vi "Configure Front Panel View.vi"(8 "error in":errorcluster, 10 "Show All":bool, 11 "Heat Flow Test Stand in":refnum<class "Heat Flow Test Stand.lvclass">) -> (0 "error out":errorcluster, 3 "Heat Flow Test Stand out":refnum<class "Heat Flow Test Stand.lvclass">)   [LabVIEW 2019, in "Test Stands.lvlib" / "Heat Flow Test Stand.lvclass"]
uses:
  Heat Flow Test Stand.lvclass
  Generic Test Stand/TS Panel Method.ctl
  Generic Test Stand/Generic Test Stand.lvclass
  Results/Results Method.ctl
  Results/Results.lvlib
  Results/DeepU Results/DeepU Results.lvclass
  DAC/DAC.lvclass
  Results/Heat Flow Results/Heat Flow Results.lvclass
  C:/Users/krio/Documents/LV_Projects/test-stand/App/Generic Test Stand/Generic Test Stand.lvclass
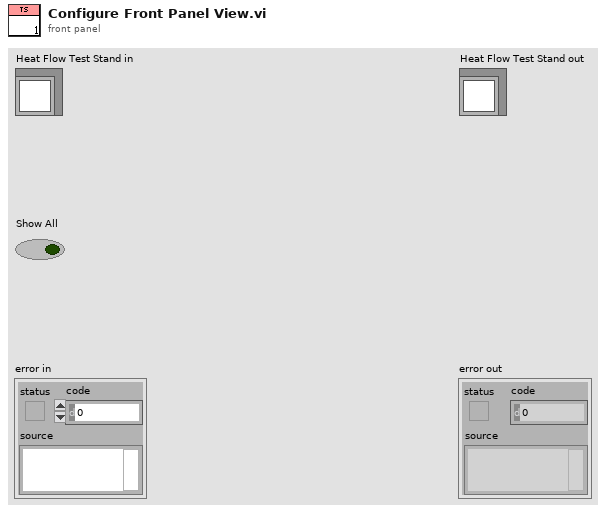
[diagram p1: front panel]
types:
  T1 = typedef "Generic Test Stand.lvclass/TS Panel Method.ctl" = enum16{"Send to Panel", "Receive from Panel", "Update Panel View"}
  T2 = typedef "Results.lvlib/Results Method.ctl" = enum16{"Get", "Set"}
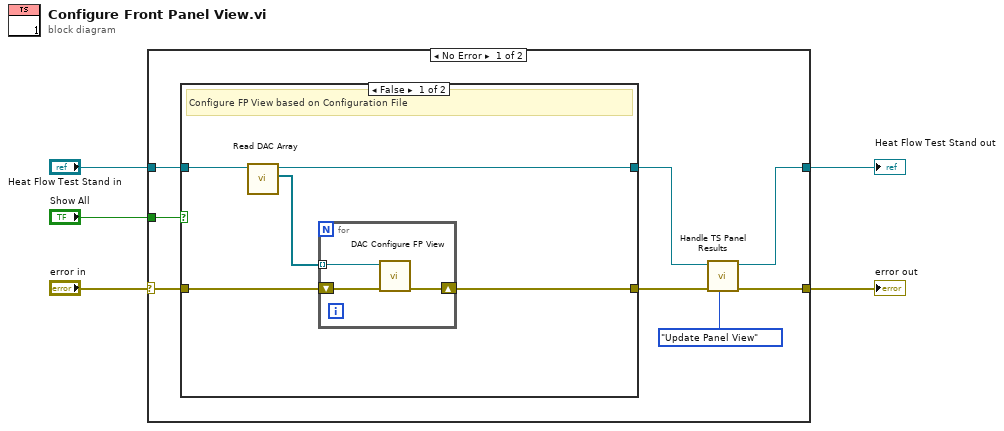
[diagram p0: block diagram]
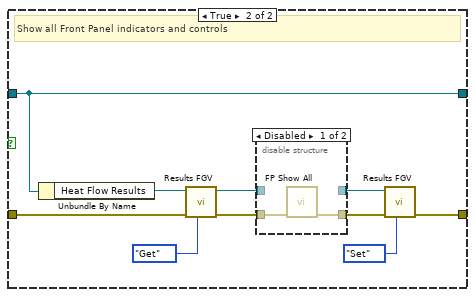
[diagram p2: hidden frame]
diagram:
  n1 = case shown="No Error" "error in" {
    selector: "error in" -> [w12 w37]
    tunnel: [w9 w37] -> w1
    tunnel: [w7 w36] -> w2
    tunnel: "Heat Flow Test Stand in" -> [w13 w36]
    tunnel: "Show All" -> [w6 _]
    frame No Error {
      n2 = case shown="False" w6 {
        tunnel: w13 -> [w18 w31]
        tunnel: w12 -> [w16 w27]
        tunnel: [w15 w24] -> w11
        tunnel: [w14 w31] -> w8
        frame False {
          # "Configure FP View based on Configuration File"
          n3 = call "Read DAC Array.vi"("Generic Test Stand in"=w18) -> ("DAC Array"=w17:refnum<class "DAC.lvclass">[], "Generic Test Stand out"=w14:refnum<class "Heat Flow Test Stand.lvclass">)  [unwired: 8 in, 1 out]
          n4 = for {
            tunnel: w17 -> [w21] mode=indexing
            shift-right: [w19] -> w15
            shift-left: w16 -> [w20]
            n5 = call-dynamic "DAC Configure FP View.vi"("error in"=w20, "DAC in"=w21) -> ("error out"=w19:errorcluster)  [unwired: 8 in, 1 out]
          }
        }
        frame True {
          # "Show all Front Panel indicators and controls"
          n6 = Unbundle By Name(w31) -> ("Heat Flow Results"=w30:refnum<class "Heat Flow Results.lvclass">)
          n7 = call-dynamic "Results FGV.vi"("Method"=Results_Method."Get", "error in"=w27, "Results in"=w30) -> ("error out"=w26:errorcluster, "Results out"=w23:refnum<class "Heat Flow Results.lvclass">)  [unwired: 7 in]
          n8 = disable-structure shown="Disabled" {
            disable-tunnel: w26 -> [w33 w34]
            disable-tunnel: [w32 w34] -> w25
            disable-tunnel: w23 -> [_ w35]
            disable-tunnel: [_ w35] -> w22
            frame Disabled {
              n9 = call "FP Show All.vi"("error in (no error)"=w33) -> ("error out"=w32:errorcluster)  [unwired: 9 in, 1 out]
            }
            frame Enabled {
            }
          }
          n10 = call-dynamic "Results FGV.vi"("Method"=Results_Method."Set", "error in"=w25, "Results in"=w22) -> ("error out"=w24:errorcluster)  [unwired: 7 in, 1 out]
        }
      }
      n11 = call-dynamic "Handle TS Panel Results.vi"("Method"=TS_Panel_Method."Update Panel View", "error in"=w11, "Heat Flow Test Stand in"=w8) -> ("error out"=w9:errorcluster, "Heat Flow Test Stand out"=w7:refnum<class "Heat Flow Test Stand.lvclass">)  [unwired: 7 in]
    }
    frame Error {
    }
  }
  "error out" <- w1
  "Heat Flow Test Stand out" <- w2
